vi "rqcBob API Test.vi"() -> ()   [LabVIEW 2019, in "rqcBob.lvclass"]
uses:
  rqcBob.lvclass
  FPGA/rqcBob/Custom Controls/Pulse Train/rqcBob Pulse Train.First Pulse Delay Mode.ctl
  Shared/Shared FPGA Lib/Shared Logic/Custom Controls/rqc Random Generator.value type.ctl
  Custom Controls/rqcBob Operation Mode.ctl
  FPGA/rqcBob/Custom Controls/Pulse Train/rqcBob Pulse Train.Generation Mode.ctl
  public/Measurements/rqcBob Read Channel Test Results.vi
panel:
  out "Detections Destribution":T1(graph)
  in  "DAC value":u16=150
  in  "DAC Value Type":T2=enum."constant"
  in  "Stop":u16
  in  "Start":u16
  in  "Close":u16=3000
  in  "Open":u16
  in  "First Pulse Delay":u16=55
  in  "First Pulse Delay Mode":T3=enum."every train"
  in  "Number of Trains":u16=4000
  in  "Number of Pulses":u16=1
  in  "Period":u16=4000
  # "Train Configuration"
  # "Modulator Configuration"
  # "Window Configuration"
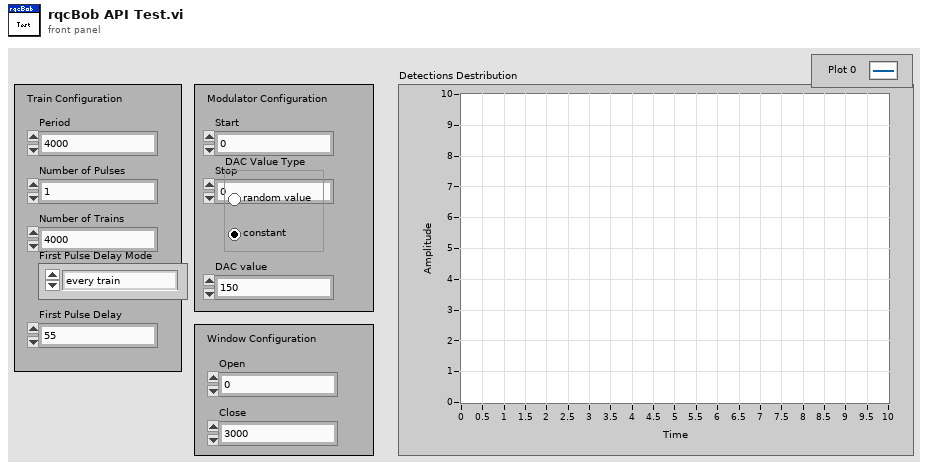
[diagram p1: front panel]
types:
  T1 = cluster{"X Values":dbl[], "Histogram: h(x)":i32[]}
  T2 = typedef "rqc Random Generator.value type.ctl" = enum32{"random value", "constant"}
  T3 = typedef "rqcBob Pulse Train.First Pulse Delay Mode.ctl" = enum8{"none", "every train", "first train"}
  T4 = typedef "rqcBob Pulse Train.Generation Mode.ctl" = enum32{"single train", "train sequence.single", "train sequence.wait for trigger", "continuous"}
  T5 = typedef "rqcBob.lvclass/rqcBob Operation Mode.ctl" = enum16{"Not Set", "Channel Test", "Key Distribution", "Modulation Level Test", "Window Test", "Delay Line Test", "Alice Modulation Level Test"}
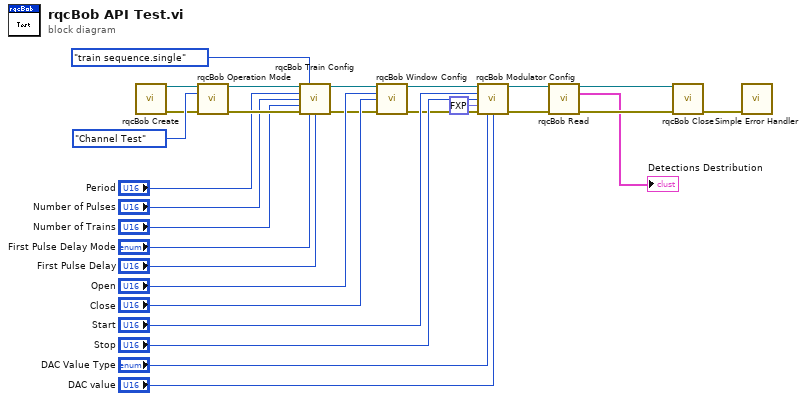
[diagram p0: block diagram]
diagram:
  n1 = call "rqcBob Create.vi"() -> ("rqcBob out"=w27:refnum<class "rqcBob.lvclass">, "error out"=w24:errorcluster)  [unwired: 14 in]
  n2 = call-dynamic "rqcBob Operation Mode.vi"("rqcBob in"=w27, "Operation Mode"=rqcBob_Operation_Mode."Channel Test", "error in (no error)"=w24) -> ("rqcBob out"=w26:refnum<class "rqcBob.lvclass">, "error out"=w22:errorcluster)  [unwired: 11 in]
  n3 = call-dynamic "rqcBob Train Config.vi"("rqcBob in"=w26, "Train.Generation Mode"=rqcBob_Pulse_Train.Generation_Mode."train sequence.single", "Train.Period"="Period", "Train.Number of Pulses"="Number of Pulses", "Train.Number of Trains"="Number of Trains", "error in (no error)"=w22, "Train.First Pulse Delay Mode"="First Pulse Delay Mode", "Train.First Pulse Delay"="First Pulse Delay") -> ("rqcBob out"=w16:refnum<class "rqcBob.lvclass">, "error out"=w13:errorcluster)  [unwired: 6 in]
  n4 = call-dynamic "rqcBob Window Config.vi"("rqcBob in"=w16, "Window.Open"="Open", "Window.Close"="Close", "error in (no error)"=w13) -> ("rqcBob out"=w12:refnum<class "rqcBob.lvclass">, "error out"=w8:errorcluster)  [unwired: 10 in]
  n5 = call-dynamic "rqcBob Modulator Config.vi"("rqcBob in"=w12, "Modulator.Start"="Start", "Modulator.Stop"="Stop", "Modulator.Clock Delay"=fxp<+,4,4> 0.0, "error in (no error)"=w8, "Modulator.Value Type"="DAC Value Type", "DAC value"="DAC value") -> ("rqcBob out"=w5:refnum<class "rqcBob.lvclass">, "error out"=w4:errorcluster)  [unwired: 7 in]
  n6 = call-poly "rqcBob Read.vi"("rqcBob in"=w5, "error in (no error)"=w4) -> ("rqcBob out"=w3:refnum<class "rqcBob.lvclass">, "Detections Destribution"=→"Detections Destribution":T1, "error out"=w2:errorcluster)  [unwired: 11 in]
  n7 = call-dynamic "rqcBob Close.vi"("rqcBob in"=w3, "error in"=w2) -> ("error out"=w28:errorcluster)  [unwired: 13 in]
  n8 = call <vilib>:"Simple Error Handler.vi"("error in (no error)"=w28) -> ()  [unwired: 4 in, 5 out]
